vi "IsFirst.vi"(8 "error in (no error)":errorcluster, 10 "Module ID":i32=-1, 11 "CloneRegRef":refnum<data-value>) -> (0 "error out":errorcluster, 1 "First?":bool, 2 "Found?":bool, 3 "CloneRegRef":refnum<data-value>)   [LabVIEW 2018, in "ModuleAdmin.lvlib" / "CloneRegistration.lvclass"]
uses:
  CloneRegistration.lvclass
  CloneRegistration.lvclass/CloneRegistration.ctl
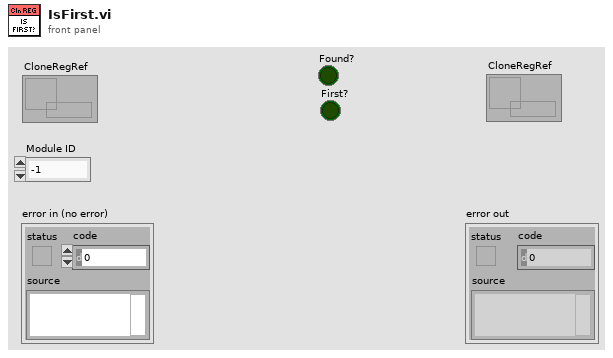
[diagram p1: front panel]
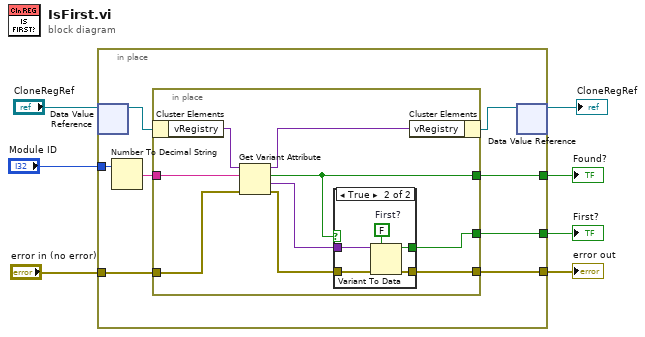
[diagram p0: block diagram]
diagram:
  n1 = in-place {
    in-place-border: "Module ID" -> [w15]
    in-place-border: [w13] -> w6
    in-place-border: [w12] -> w5
    in-place-border: [w11] -> w4
    in-place-border: "error in (no error)" -> [w10]
    n2 = in-place-dvr #1("CloneRegRef") -> (w9:refnum<class "CloneRegistration.lvclass">)  [unwired: 1 out]
    n3 = Number To Decimal String(number=w15) -> (decimal integer string=w14:string)  [unwired: 1 in]
    n4 = in-place {
      in-place-border: w14 -> [w24]
      in-place-border: [w22] -> w13
      in-place-border: [w19] -> w12
      in-place-border: [w18] -> w11
      in-place-border: w10 -> [w17]
      n5 = in-place-cluster #2(w9) -> ("vRegistry"=w23:variant)
      n6 = Get Variant Attribute(Variant=w23, name=w24, error in=w17) -> (duplicate Variant=w16:variant, found=w22:bool, value=w21:variant, error out=w20:errorcluster)  [unwired: 1 in]
      n7 = case shown="True" w22 {
        tunnel: w21 -> [_ w30]
        tunnel: w20 -> [w25 w29]
        tunnel: [_ w27] -> w19
        tunnel: [w25 w26] -> w18
        frame False {
        }
        frame True {
          w28 = FALSE  # First?
          n8 = Variant To Data(error in=w29, type=w28, Variant=w30) -> (data=w27:bool, error out=w26:errorcluster)
        }
      }
      n9 = in-place-cluster #2("vRegistry"=w16) -> (w8:refnum<class "CloneRegistration.lvclass">)
    }
    n10 = in-place-dvr #1(w8) -> (→"CloneRegRef":refnum<data-value>)  [unwired: 1 out]
  }
  "error out" <- w4
  "Found?" <- w6
  "First?" <- w5
